vi "accept_connection.vi"(4 "WebSocket Logger":refnum<class "WebSocket Logger.lvclass">, 6 "Sec-WebSocket-Protocol":string[](array[string]), 8 "error in (no error)":errorcluster, 9 "remote address":string, 10 "remote port":u16, 11 "WebSocket Echo Server in":refnum<class "WebSocket Echo Server.lvclass">) -> (0 "error out":errorcluster, 1 "accept connection?":bool, 2 "Sec-WebSocket-Protocol accepted":string, 3 "WebSocket Echo Server out":refnum<class "WebSocket Echo Server.lvclass">)   [LabVIEW 2019, in "WebSocket Echo Server.lvclass"]
uses:
  WebSocket Echo Server.lvclass
  TauTerra WebSocketServer Toolkit.lvlibp/classes/WebSocket Logger/WebSocket Logger.lvclass
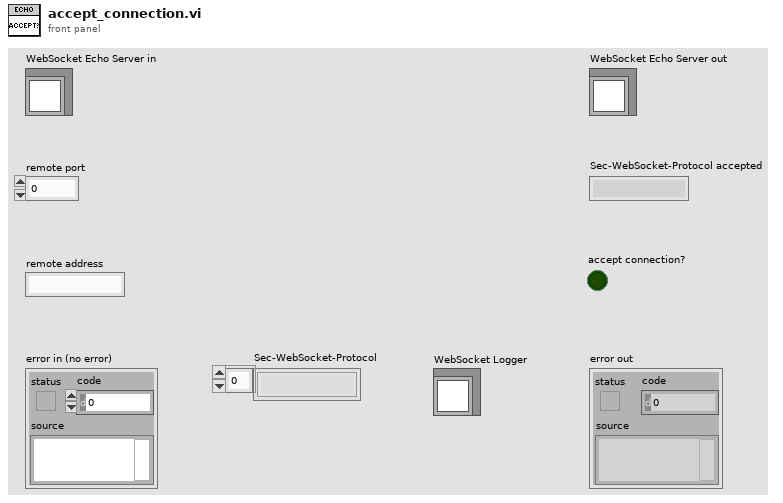
[diagram p1: front panel]
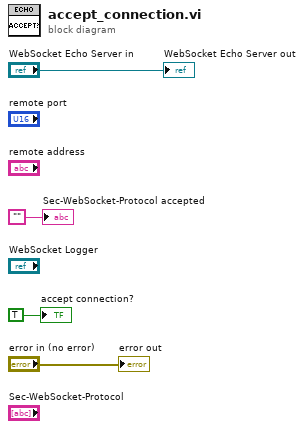
[diagram p0: block diagram]
diagram:
  "error out" <- "error in (no error)"
  "WebSocket Echo Server out" <- "WebSocket Echo Server in"
  "Sec-WebSocket-Protocol accepted" <- ""
  "accept connection?" <- TRUE ("accept connection?")
